vi "GT_Start.vi"(2 "mask":i16, 3 "rtn_In":cluster{"rtn":i16, "Func":string}) -> (1 "rtn_Out":cluster{"rtn":i16, "Func":string})   [LabVIEW 2014]
uses:
  axxon_Gold.vi
  VC6/gts.dll
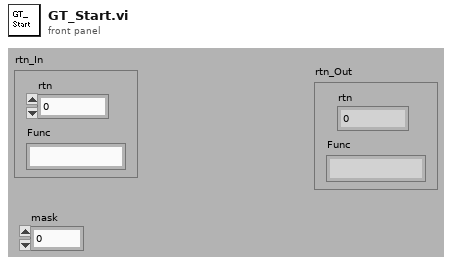
[diagram p1: front panel]
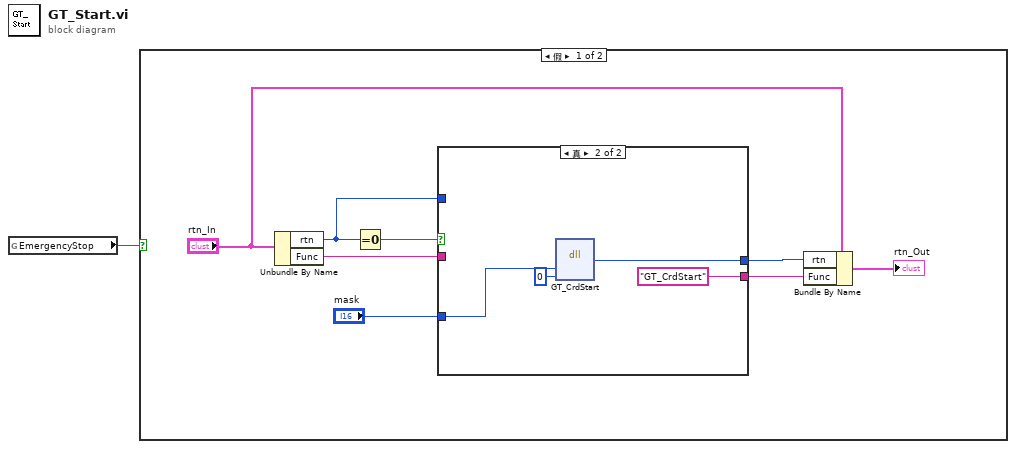
[diagram p0: block diagram]
diagram:
  n1 = global read "axxon_Gold.vi" "EmergencyStop"() -> (w1:bool)
  n2 = case shown="假" w1 {
    frame False {
      n3 = Unbundle By Name("rtn_In") -> ("rtn"=w3:i16, "Func"=w2:string)
      n4 = Equal To 0?(x=w3) -> (x = 0?=w9:bool)
      n5 = case shown="真" w9 {
        tunnel: [w11 w15] -> w7
        tunnel: [w10 "GT_CrdStart" ("Func")] -> w6
        tunnel: "mask" -> [_ w13]
        tunnel: w3 -> [w11 _]
        tunnel: w2 -> [w10 _]
        frame False {
        }
        frame True {
          n6 = dll-call lib="PTH2Fabs DNewGTS AC-800LWin7版源程序-20170926gts85VC6gts.dll" fn="GT_CrdStart"("mask"=w13, "Option"=i16 0) -> ("rtn"=w15:i16)  [unwired: 5 in, 2 out]
        }
      }
      n7 = Bundle By Name(cluster="rtn_In", "rtn"=w7, "Func"=w6) -> (→"rtn_Out":cluster{"rtn":i16, "Func":string})
    }
    frame True {
    }
  }
